vi "Pre-Actor.vi"(8 "error in":errorcluster, 11 "PowerSupply in":refnum<class "PowerSupply.lvclass">) -> (0 "error out":errorcluster, 3 "PowerSupply out":refnum<class "PowerSupply.lvclass">)   [LabVIEW 2019, in "PowerSupply.lvlib" / "PowerSupply.lvclass"]
doc: "This override VI is to provide the means for children classes to perform application specific post launch initialization functions that must be performed *prior* to calling the actor."
uses:
  Library/PowerSupply.lvclass
  Library/PowerSupply.lvclass/PowerSupply.ctl
  builds/Instruments/Instruments.lvlibp/Library/Instruments.lvclass
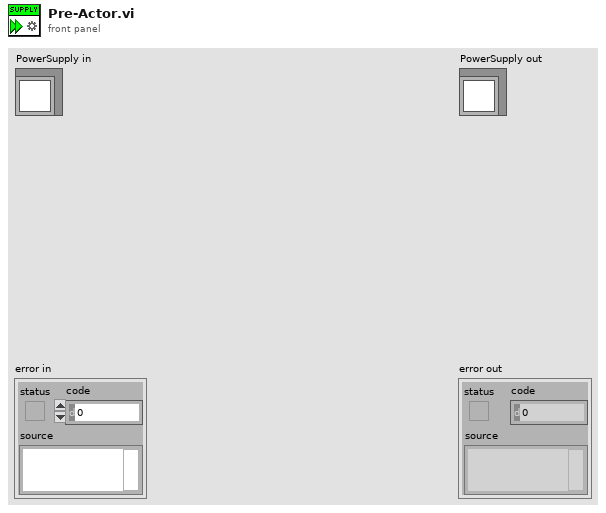
[diagram p1: front panel]
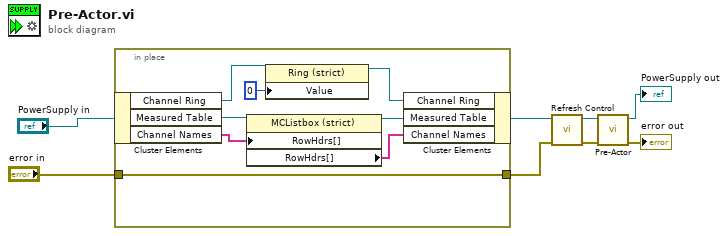
[diagram p0: block diagram]
diagram:
  n1 = in-place {
    in-place-border: "error in" -> [w12]
    in-place-border: [w12] -> w3
    n2 = in-place-cluster #1("PowerSupply in") -> ("Channel Ring"=w11:refnum<vi>, "Measured Table"=w16:refnum<vi>, "Channel Names"=w14:string[])
    n3 = property class="MCListbox (strict)"(reference=w16, "RowHdrs[]"=w14) -> (reference out=w15:refnum<vi>, "RowHdrs[]"=w13:string[])  [unwired: 1 in, 1 out]
    n4 = property class="Ring (strict)"(reference=w11, "Value"=u16 0) -> (reference out=w10:refnum<vi>)  [unwired: 1 in, 1 out]
    n5 = in-place-cluster #1("Channel Ring"=w10, "Measured Table"=w15, "Channel Names"=w13) -> (w4:refnum<class "PowerSupply.lvclass">)
  }
  n6 = call "Refresh Control.vi"("error in"=w3, "PowerSupply in"=w4) -> ("error out"=w1:errorcluster, "PowerSupply out"=w2:refnum<class "PowerSupply.lvclass">)  [unwired: 8 in]
  n7 = call-parent "Pre-Actor.vi"("error in (no error)"=w1, "Instruments in"=w2) -> ("error out"=→"error out":errorcluster, "Instruments out"=→"PowerSupply out":refnum<class "PowerSupply.lvclass">)  [unwired: 8 in]
